vi "Default selector.vi"(8 "error in":errorcluster, 11 "Car wash data":T1 {"Elapsed Time" format="%0.2f"}) -> (0 "error out":errorcluster, 3 "output cluster":T1 {"Elapsed Time" format="%0.2f"})   [LabVIEW 2015]
uses:
  controls/Car wash data.ctl
  USB Template (LV 8.6)/Car Wash/Controls/Wash Options.ctl
  USB Template (LV 8.6)/Car Wash/Controls/Car Wash Indicators.ctl
  controls/times.ctl
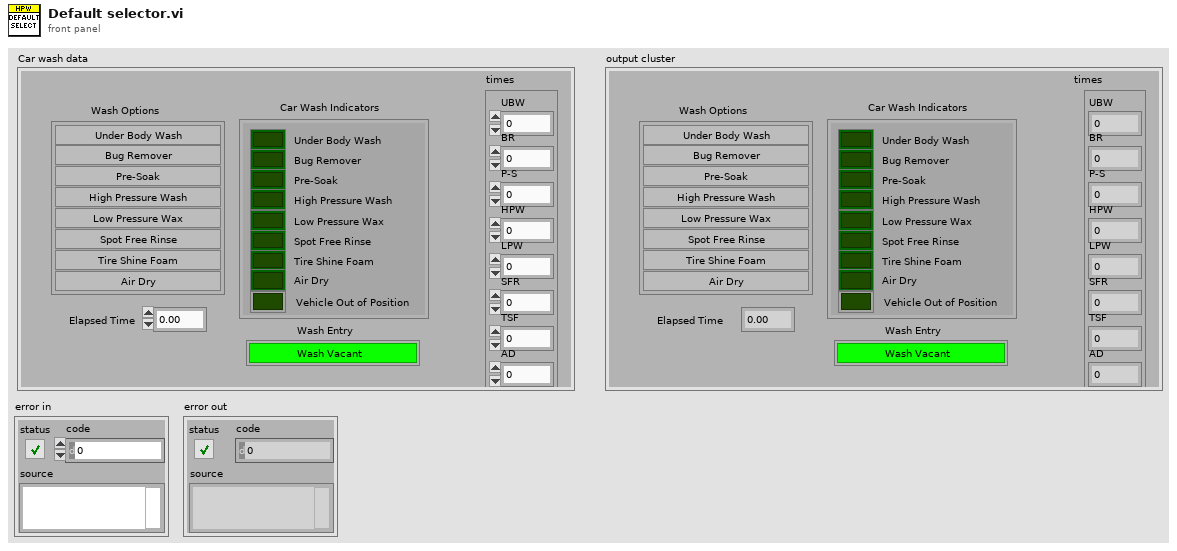
[diagram p1: front panel]
types:
  T1 = typedef "Car wash data.ctl" = cluster{"Wash Options":T2, "Car Wash Indicators":T3, "Wash Entry":bool, "Elapsed Time":dbl, "times":T4}
  T2 = typedef "Wash Options.ctl" = cluster{"Underbody Wash":bool, "Bug Remover":bool, "Pre-Soak":bool, "High Pressure Wash":bool, "Low Pressure Wax":bool, "Spot Free Rinse":bool, "Tire Shine Foam":bool, "Air Dry":bool}
  T3 = typedef "Car Wash Indicators.ctl" = cluster{"Under Body Wash":bool, "Bug Remover":bool, "Pre-Soak":bool, "High Pressure Wash":bool, "Low Pressure Wax":bool, "Spot Free Rinse":bool, "Tire Shine Foam":bool, "Air Dry":bool, "Vehicle Out of Position":bool}
  T4 = typedef "times.ctl" = cluster{"UBW":dbl, "BR":dbl, "P-S":dbl, "HPW":dbl, "LPW":dbl, "SFR":dbl, "TSF":dbl, "AD":dbl}
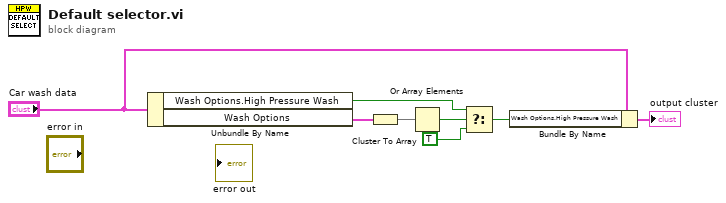
[diagram p0: block diagram]
diagram:
  n1 = Unbundle By Name("Car wash data") -> ("Wash Options.High Pressure Wash"=w4:bool, "Wash Options"=w1:T2)
  n2 = Cluster To Array(cluster=w1) -> (array=w2:bool[])
  n3 = Or Array Elements(Boolean array=w2) -> (logical OR=w3:bool)
  n4 = Select(t=w4, s=w3, f=TRUE) -> (s? t:f=w7:bool)
  n5 = Bundle By Name(cluster="Car wash data", "Wash Options.High Pressure Wash"=w7) -> (→"output cluster":T1)
